vi "FlatToRichrfcontrol_GetRFTileSampleRateRequest.vi"(5 "OutputClusterType":T1, 11 "InputCluster":T3) -> (3 "OutputCluster":T1)   [LabVIEW 2024, in "FlexSDR_gRPC_client.lvlib"]
uses:
  rfcontrol_GetRFTileSampleRateRequest_Flat.ctl
  rfcontrol_RFTile.ctl
  rfcontrol_GetRFTileSampleRateRequest.ctl
  FlexSDR_gRPC_client.lvlib
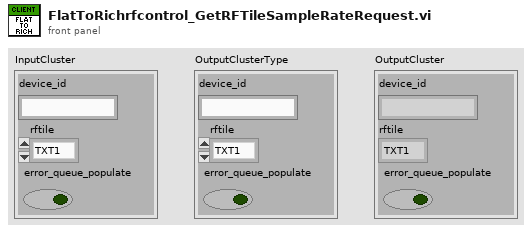
[diagram p1: front panel]
types:
  T1 = typedef "FlexSDR_gRPC_client.lvlib/rfcontrol_GetRFTileSampleRateRequest.ctl" = cluster{"device_id":string, "rftile":T2, "error_queue_populate":bool}
  T2 = typedef "FlexSDR_gRPC_client.lvlib/rfcontrol_RFTile.ctl" = enum32{"TXT1", "TXT2", "RXT1", "RXT2", "WRXT"}
  T3 = typedef "FlexSDR_gRPC_client.lvlib/rfcontrol_GetRFTileSampleRateRequest_Flat.ctl" = cluster{"device_id":string, "rftile":T2, "error_queue_populate":bool}
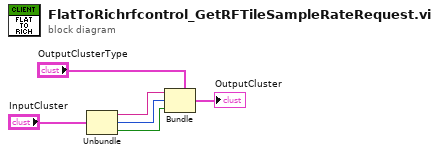
[diagram p0: block diagram]
diagram:
  n1 = Unbundle "Unbundle"("InputCluster") -> ("device_id"=w3:string, "rftile"=w2:T2, "error_queue_populate"=w1:bool)
  n2 = Bundle "Bundle"(cluster="OutputClusterType", "device_id"=w3, "rftile"=w2, "error_queue_populate"=w1) -> (→"OutputCluster":T1)
